vi "Steering Motor Write.vi"(6 "Configuration":T3={"Accelerometer Bias"={"X (m/s)"=0.0, "Y (m/s)"=0.0, "Z (m/s)"=0.0}, "Gyroscope Bias"={"X (m/s)"=0.0, "Y (m/s)"=0.0, "Z (m/s)"=0.0}, "Steering Motor Gear Ratio"=611.0, "Steering Pully Gear Ratio"=1.0, "Steering Encoder CPR"=1024.0, "Steering Motor Max RPM"=4000.0, "Wheelbase (m)"=1.12, "Fork Angle (rad)"=1.3, "Balancing Controller"={"Kp (/s)"=0.0, "Kd (1)"=0.0}, "Max Allowed Steering Angle (rad)"=0.7, "Task Periods"={"Emergency Stop (us)"=0, "IMU (us)"=0, "Steering Motor Encoder (us)"=0, "State Estimator (us)"=0, "Balancing Controller (us)"=0, "GNSS (us)"=0, "Logging (us)"=0, "Drive Motor (us)"=0}, "Drive Motor Gear Ratio"=0.7, "lr"=0.0, "lf"=0.0, "lambda"=0.0, "k1"=0.0, "k2"=0.0, "e1_max"=0.0, "Ad_t"=0.0, "Bd_t"=0.0, "C_t"=0.0, "D_t"=0.0, "Initialization"=[0.0, 0.0, 0.0, 0.0, 0.0, 0.0, 0.0]}, 8 "Controller Data In":refnum<data-value>, 9 "Steering Angle Rate (rad/s)":dbl, 10 "Steering Motor Handle In":T2, 11 "Error In":errorcluster) -> (0 "Controller Data Out":refnum<data-value>, 1 "Steering Motor Data":T1, 2 "Steering Motor Handle Out":T2, 3 "Error Out":errorcluster)   [LabVIEW 2021]
uses:
  Configuration/Configuration.ctl
  Steering Motor Handle.ctl
  Steering Motor Data.ctl
  Logging/Controller Data.ctl
  Drive Motor/Drive Motor Data.ctl
  <vilib>/myRIO/Instrument Drivers/Onboard IO/PWM/typedefs/PWM Reference.ctl
  <vilib>/myRIO/Common/Instrument Driver Framework/Utilities/typedefs/myRIO Generic Hardware Reference.ctl
  <vilib>/myRIO/Common/Instrument Driver Framework/Utilities/typedefs/Hardware Version Enum.ctl
  <vilib>/myRIO/Common/Instrument Driver Framework/Utilities/typedefs/myRIO v1.0 Reference.ctl
  <vilib>/myRIO/Common/Instrument Driver Framework/Utilities/typedefs/Generic FPGA Reference.ctl
  <vilib>/myRIO/Common/Instrument Driver Framework/myRIO v1.0/PWM/typedefs/PWM Channels Enum.ctl
  <vilib>/myRIO/Instrument Drivers/Onboard IO/PWM/typedefs/PWM Configuration.ctl
  <vilib>/userDefined/High Color/nirio_resource_hc.ctl
  <vilib>/myRIO/Common/Instrument Driver Framework/Utilities/vis/Is FPGA Ref Available.vi
  <vilib>/myRIO/Common/Instrument Driver Framework/myRIO v1.0/PWM/vis/myRIO v1.1 Open PWM.vi
  <vilib>/myRIO/Instrument Drivers/Onboard IO/PWM/vis/Set Duty Cycle and Frequency.vi
  <vilib>/myRIO/Common/Instrument Driver Framework/Utilities/vis/Validate Channels.vi
  <vilib>/myRIO/Common/Instrument Driver Framework/myRIO v1.0/PWM/vis/myRIO v1.0 Reserve PWM.vi
  <vilib>/myRIO/Common/Instrument Driver Framework/myRIO v1.0/PWM/vis/myRIO v1.0 Build MUX Configuration PWM.vi
  <vilib>/myRIO/Common/Instrument Driver Framework/myRIO v1.0/Resource Manager/vis/myRIO v1.0 Reserve Channel List.vi
  <vilib>/myRIO/Common/Instrument Driver Framework/myRIO v1.0/Resource Manager/vis/myRIO v1.0 Create Configuration List.vi
  <vilib>/myRIO/Common/Instrument Driver Framework/myRIO v1.0/Resource Manager/vis/myRIO v1.0 Reserve Channel.vi
  <vilib>/myRIO/Common/Instrument Driver Framework/myRIO v1.0/Resource Manager/vis/myRIO v1.0 Unreserve Channel.vi
  <vilib>/myRIO/Common/Instrument Driver Framework/myRIO v1.0/Resource Manager/vis/myRIO v1.0 Build Mutex Name.vi
  <vilib>/Utility/VariantDataType/GetNumericInfo.vi
  <vilib>/Utility/error.llb/Error Cluster From Error Code.vi
  <vilib>/myRIO/Common/Instrument Driver Framework/myRIO v1.0/myRIO v1.1 Open.vi
  <vilib>/myRIO/Common/Instrument Driver Framework/Utilities/vis/IO Manager.vi
  <vilib>/myRIO/Common/Instrument Driver Framework/Utilities/vis/Configuration Manager.vi
  <vilib>/myRIO/Common/Instrument Driver Framework/myRIO v1.0/Resource Manager/vis/myRIO v1.0 Configure IO.vi
  <vilib>/myRIO/Common/Instrument Driver Framework/myRIO v1.0/myRIO v1.0 Close.vi
  <vilib>/myRIO/Common/Instrument Driver Framework/myRIO v1.0/PWM/vis/myRIO v1.0 Write PWM.vi
  <vilib>/myRIO/Express VI/Onboard IO/PWM/PWM Express VI.xnode
  <vilib>/myRIO/Instrument Drivers/Onboard IO/PWM/vis/myRIO PWM Open.xnode
  <vilib>/myRIO/Instrument Drivers/Onboard IO/PWM/PWM.lvlib
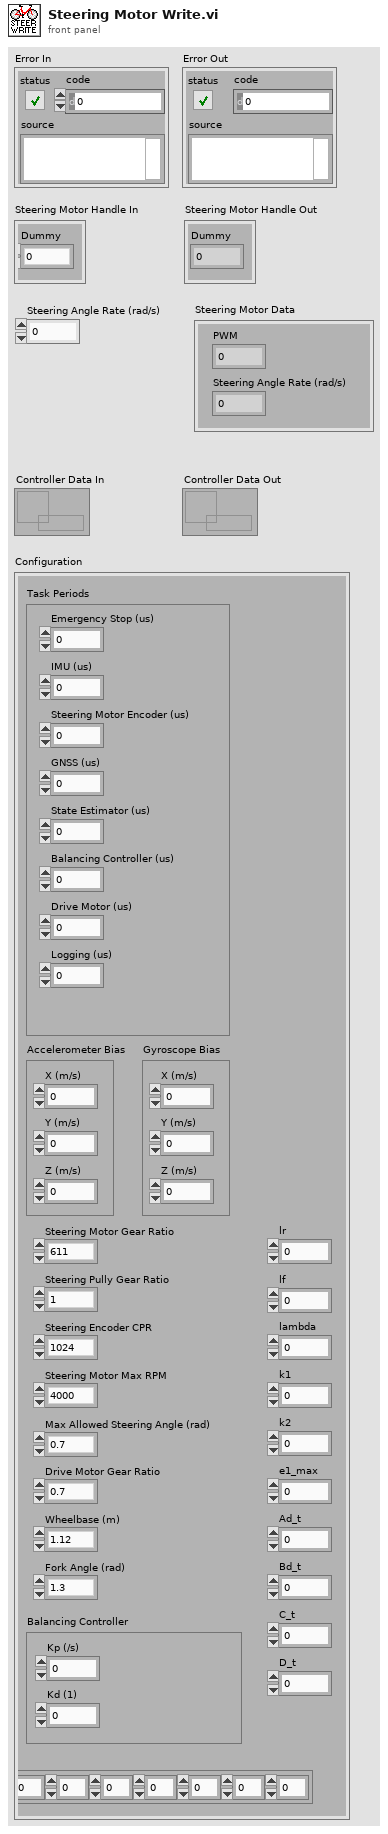
[diagram p1: front panel]
types:
  T1 = typedef "Steering Motor Data.ctl" = cluster{"PWM":dbl, "Steering Angle Rate (rad/s)":dbl}
  T2 = typedef "Steering Motor Handle.ctl" = cluster{"Dummy":dbl}
  T3 = typedef "Configuration.ctl" = cluster{"Accelerometer Bias":cluster{"X (m/s)":dbl, "Y (m/s)":dbl, "Z (m/s)":dbl}, "Gyroscope Bias":cluster{"X (m/s)":dbl, "Y (m/s)":dbl, "Z (m/s)":dbl}, "Steering Motor Gear Ratio":dbl, "Steering Pully Gear Ratio":dbl, "Steering Encoder CPR":dbl, "Steering Motor Max RPM":dbl, "Wheelbase (m)":dbl, "Fork Angle (rad)":dbl, "Balancing Controller":cluster{"Kp (/s)":dbl, "Kd (1)":dbl}, "Max Allowed Steering Angle (rad)":dbl, "Task Periods":cluster{"Emergency Stop (us)":i64, "IMU (us)":i64, "Steering Motor Encoder (us)":i64, "State Estimator (us)":i64, "Balancing Controller (us)":i64, "GNSS (us)":i64, "Logging (us)":i64, "Drive Motor (us)":i64}, "Drive Motor Gear Ratio":dbl, "lr":dbl, "lf":dbl, "lambda":dbl, "k1":dbl, "k2":dbl, "e1_max":dbl, "Ad_t":dbl, "Bd_t":dbl, "C_t":dbl, "D_t":dbl, "Initialization":dbl[]}
  T4 = typedef "Controller Data.ctl" = cluster{"Drive Motor Data":T5, "Steering Motor Data":T1}
  T5 = typedef "Drive Motor Data.ctl" = cluster{"Angular Speed (rad/s)":dbl, "Input Current (A)":dbl, "Motor Current (A)":dbl, "MOSFET Temperature (deg C)":dbl}
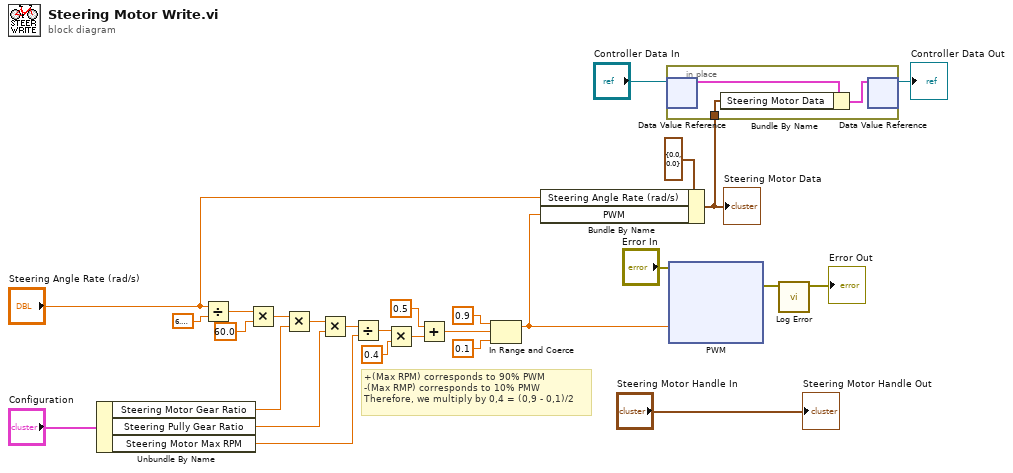
[diagram p0: block diagram]
diagram:
  # "+(Max RPM) corresponds to 90% PWM\n-(Max RMP) corresponds to 10% PMW\nTherefore, we multiply by 0,4 = (0,9 - 0,1)/2"
  n1 = Unbundle By Name("Configuration") -> ("Steering Motor Gear Ratio"=w19:dbl, "Steering Pully Gear Ratio"=w20:dbl, "Steering Motor Max RPM"=w17:dbl)
  n2 = Divide(x="Steering Angle Rate (rad/s)", y=6.283185307179586) -> (x/y=w25:dbl)
  n3 = Multiply(x=w25, y=60.0) -> (x*y=w22:dbl)
  n4 = Multiply(x=w22, y=w19) -> (x*y=w21:dbl)
  n5 = Multiply(x=w21, y=w20) -> (x*y=w18:dbl)
  n6 = Divide(x=w18, y=w17) -> (x/y=w12:dbl)
  n7 = Multiply(x=w12, y=0.4) -> (x*y=w9:dbl)
  n8 = Add(x=0.5 ("y"), y=w9) -> (x+y=w16:dbl)
  n9 = In Range and Coerce(upper limit=0.9, x=w16, lower limit=0.1) -> (coerced(x)=w5:dbl)  [unwired: 1 out]
  n10 = Bundle By Name(cluster=T1 {"PWM"=0.0, "Steering Angle Rate (rad/s)"=0.0} ("Steering Motor Data"), "Steering Angle Rate (rad/s)"="Steering Angle Rate (rad/s)", "PWM"=w5) -> (w1:T1)
  "Steering Motor Data" <- w1
  n11 = in-place {
    in-place-border: w1 -> [w28]
    n12 = in-place-dvr #1("Controller Data In") -> (w30:T4)  [unwired: 1 out]
    n13 = Bundle By Name(cluster=w30, "Steering Motor Data"=w28) -> (w29:T4)
    n14 = in-place-dvr #1(w29) -> (→"Controller Data Out":refnum<data-value>)  [unwired: 1 out]
  }
  n15 = xnode "PWM"("Duty Cycle"=w5, "error in (no error)"="Error In") -> ("error out"=w8:errorcluster)
  n16 = call "Log Error.vi"("Error In"=w8) -> ("Error Out"=→"Error Out":errorcluster)  [unwired: 10 in]
  "Steering Motor Handle Out" <- "Steering Motor Handle In"
